vi "CRYSet Calibration Step to Calibrated Device.vi"(11 "Calibration setup In":string) -> (2 "output Calibration":T4 {"Calibration 2D"."Sens Curve"."Z data" items=["dB", "Lin"]; "Calibration 2D"."Sens Curve"."X data" items=["dB", "Lin"]; "Calibration 2D"."Sens Curve"."Y data" items=["dB", "Lin"]; "Calibration 2D"."Sens Curve"."Z dB ref" format="%.1f"; "Calibration 2D"."Sens Curve"."Z axis" items=["Log", "Lin"]; "Calibration 2D"."Sens Curve"."X dB ref" format="%.1f"; "Calibration 2D"."Sens Curve"."X axis" items=["Log", "Lin"]; "Calibration 2D"."Sens Curve"."Y axis" items=["Log", "Lin"]; "Calibration 2D"."Sens Curve"."Y dB ref" format="%.1f"; "Calibration 2D"."Sens Curve"."Curve"."z" format="%.2f"; "Calibration 2D"."Sens Curve"."Curve"."y" format="%.2f"; "Calibration 2D"."Sens Curve"."Curve"."x" format="%.2f"; "Calibration 2D"."EQ Curve"."Z data" items=["dB", "Lin"]; "Calibration 2D"."EQ Curve"."X data" items=["dB", "Lin"]; "Calibration 2D"."EQ Curve"."Y data" items=["dB", "Lin"]; "Calibration 2D"."EQ Curve"."Z dB ref" format="%.1f"; "Calibration 2D"."EQ Curve"."Z axis" items=["Log", "Lin"]; "Calibration 2D"."EQ Curve"."X dB ref" format="%.1f"; "Calibration 2D"."EQ Curve"."X axis" items=["Log", "Lin"]; "Calibration 2D"."EQ Curve"."Y axis" items=["Log", "Lin"]; "Calibration 2D"."EQ Curve"."Y dB ref" format="%.1f"; "Calibration 2D"."EQ Curve"."Curve"."z" format="%.2f"; "Calibration 2D"."EQ Curve"."Curve"."y" format="%.2f"; "Calibration 2D"."EQ Curve"."Curve"."x" format="%.2f"; "Calibration 2D"."Corr Curve"."Z data" items=["dB", "Lin"]; "Calibration 2D"."Corr Curve"."X data" items=["dB", "Lin"]; "Calibration 2D"."Corr Curve"."Y data" items=["dB", "Lin"]; "Calibration 2D"."Corr Curve"."Z dB ref" format="%.1f"; "Calibration 2D"."Corr Curve"."Z axis" items=["Log", "Lin"]; "Calibration 2D"."Corr Curve"."X dB ref" format="%.1f"; "Calibration 2D"."Corr Curve"."X axis" items=["Log", "Lin"]; "Calibration 2D"."Corr Curve"."Y axis" items=["Log", "Lin"]; "Calibration 2D"."Corr Curve"."Y dB ref" format="%.1f"; "Calibration 2D"."Corr Curve"."Curve"."z" format="%.2f"; "Calibration 2D"."Corr Curve"."Curve"."y" format="%.2f"; "Calibration 2D"."Corr Curve"."Curve"."x" format="%.2f"; "Calibration 2D"."Calibration"."EQ Step size" items=["R10", "R20", "R40", "R80", "User"]; "Calibration 2D"."Calibration"."Corr Step size" items=["R10", "R20", "R40", "R80", "User"]}, 3 "Calibration flattened out":string)   [LabVIEW 2013]
uses:
  Typedef Control/CRYCalibration All Cluster.ctl
  Typedef Control/CRYCalibration 2DCluster.ctl
  Typedef Control/CRYCalibration Cluster.ctl
  Typedef Control/CRYData Cluster.ctl
  CRYMainGlobal.vi
panel:
  in  "Calibration 2D":T1[](array[typedef]) {"Sens Curve"."Z data" items=["dB", "Lin"]; "Sens Curve"."X data" items=["dB", "Lin"]; "Sens Curve"."Y data" items=["dB", "Lin"]; "Sens Curve"."Z dB ref" format="%.1f"; "Sens Curve"."Z axis" items=["Log", "Lin"]; "Sens Curve"."X dB ref" format="%.1f"; "Sens Curve"."X axis" items=["Log", "Lin"]; "Sens Curve"."Y axis" items=["Log", "Lin"]; "Sens Curve"."Y dB ref" format="%.1f"; "Sens Curve"."Curve"."z" format="%.2f"; "Sens Curve"."Curve"."y" format="%.2f"; "Sens Curve"."Curve"."x" format="%.2f"; "EQ Curve"."Z data" items=["dB", "Lin"]; "EQ Curve"."X data" items=["dB", "Lin"]; "EQ Curve"."Y data" items=["dB", "Lin"]; "EQ Curve"."Z dB ref" format="%.1f"; "EQ Curve"."Z axis" items=["Log", "Lin"]; "EQ Curve"."X dB ref" format="%.1f"; "EQ Curve"."X axis" items=["Log", "Lin"]; "EQ Curve"."Y axis" items=["Log", "Lin"]; "EQ Curve"."Y dB ref" format="%.1f"; "EQ Curve"."Curve"."z" format="%.2f"; "EQ Curve"."Curve"."y" format="%.2f"; "EQ Curve"."Curve"."x" format="%.2f"; "Corr Curve"."Z data" items=["dB", "Lin"]; "Corr Curve"."X data" items=["dB", "Lin"]; "Corr Curve"."Y data" items=["dB", "Lin"]; "Corr Curve"."Z dB ref" format="%.1f"; "Corr Curve"."Z axis" items=["Log", "Lin"]; "Corr Curve"."X dB ref" format="%.1f"; "Corr Curve"."X axis" items=["Log", "Lin"]; "Corr Curve"."Y axis" items=["Log", "Lin"]; "Corr Curve"."Y dB ref" format="%.1f"; "Corr Curve"."Curve"."z" format="%.2f"; "Corr Curve"."Curve"."y" format="%.2f"; "Corr Curve"."Curve"."x" format="%.2f"; "Calibration"."EQ Step size" items=["R10", "R20", "R40", "R80", "User"]; "Calibration"."Corr Step size" items=["R10", "R20", "R40", "R80", "User"]}
  in  "Hz Out":dbl caption="Hz"
  in  "dB Out":dbl caption="Sensitivity" format="%#.2g"
  in  "Sens unit Out":string="V/V"
  out "EQ Curve Out":string caption="均等化曲线"
  out "dB ref Out":dbl=1.0 caption="dB参考" format="%#_3p"
  out "unit Out":string="V" caption="单位"
  in  "Sensitivity Out":dbl=1e-50 caption="感度" min=1e-50 format="%#_6p"
  out "Sens Value Out":string caption="感度值"
  out "Corre Curve Out":string caption="修正曲线"
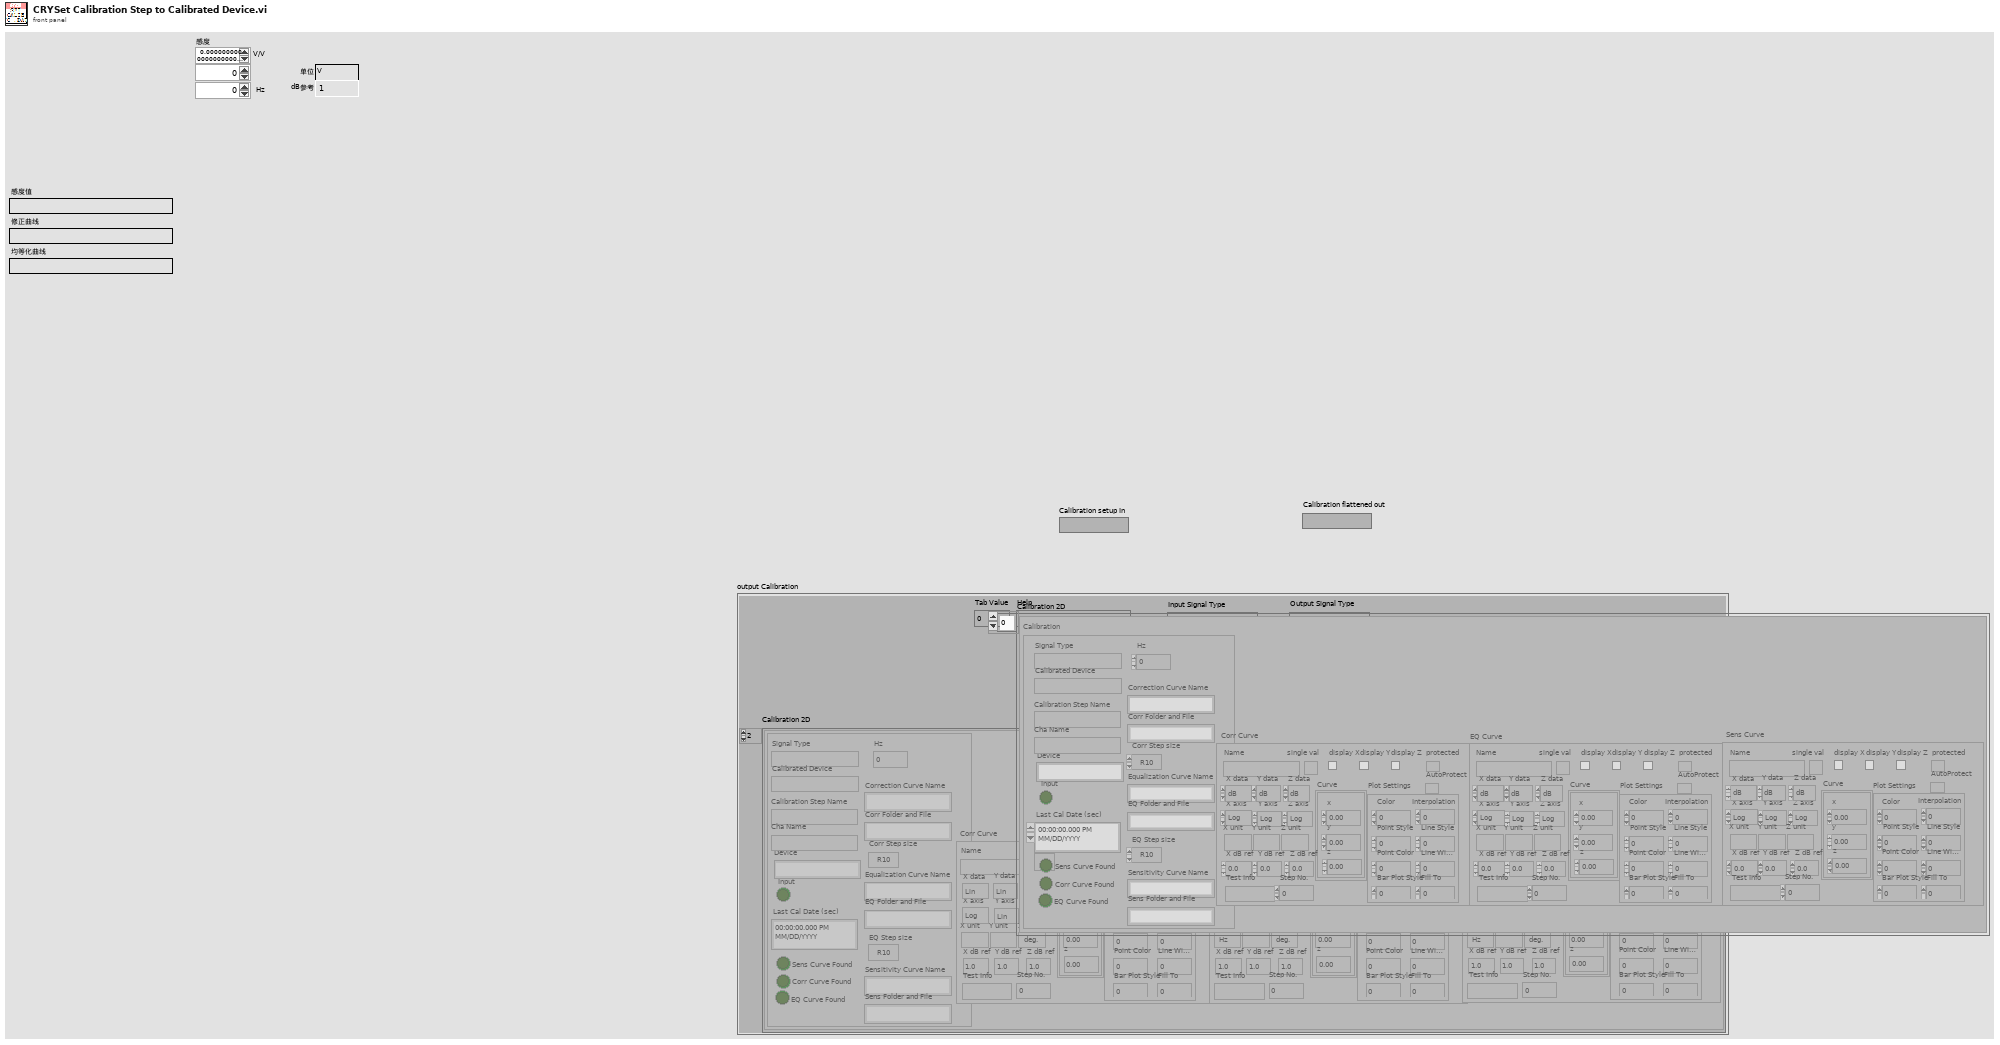
[diagram p1: front panel]
types:
  T1 = typedef "CRYCalibration 2DCluster.ctl" = cluster{"Calibration":T2, "Corr Curve":T3, "EQ Curve":T3, "Sens Curve":T3}
  T2 = typedef "CRYCalibration Cluster.ctl" = cluster{"Calibration Step Name":string, "Device":string, "Correction Curve Name":string, "Equalization Curve Name":string, "Sensitivity Curve Name":string, "Corr Folder and File":string, "EQ Folder and File":string, "Sens Folder and File":string, "Corr Step size":u16, "EQ Step size":u16, "Input":bool, "Last Cal Date (sec)":timestamp, "Cha Name":string, "Corr Curve Found":bool, "EQ Curve Found":bool, "Sens Curve Found":bool, "Signal Type":string, "Calibrated Device":string, "Hz":u32}
  T3 = typedef "CRYData Cluster.ctl" = cluster{"Name":string, "Curve":cluster{"x":dbl, "y":dbl, "z":dbl}[], "X data":u16, "Y data":u16, "Z data":u16, "X axis":u16, "Y axis":u16, "Z axis":u16, "X unit":string, "Y unit":string, "Z unit":string, "X dB ref":dbl, "Y dB ref":dbl, "Z dB ref":dbl, "single val":bool, "protected":bool, "display X":bool, "display Y":bool, "display Z":bool, "Test Info":string, "Step No.":i32, "Plot Settings":cluster{"Color":u32, "Interpolation":u8, "Point Style":u8, "Line Style":u8, "Point Color":u32, "Line Width":u8, "Bar Plot Style":u8, "Fill To":i16}, "AutoProtect":bool}
  T4 = typedef "CRYCalibration All Cluster.ctl" = cluster{"Calibration 2D":T1[], "Help":string, "Tab Value":i32, "Input Signal Type":string, "Output Signal Type":string}
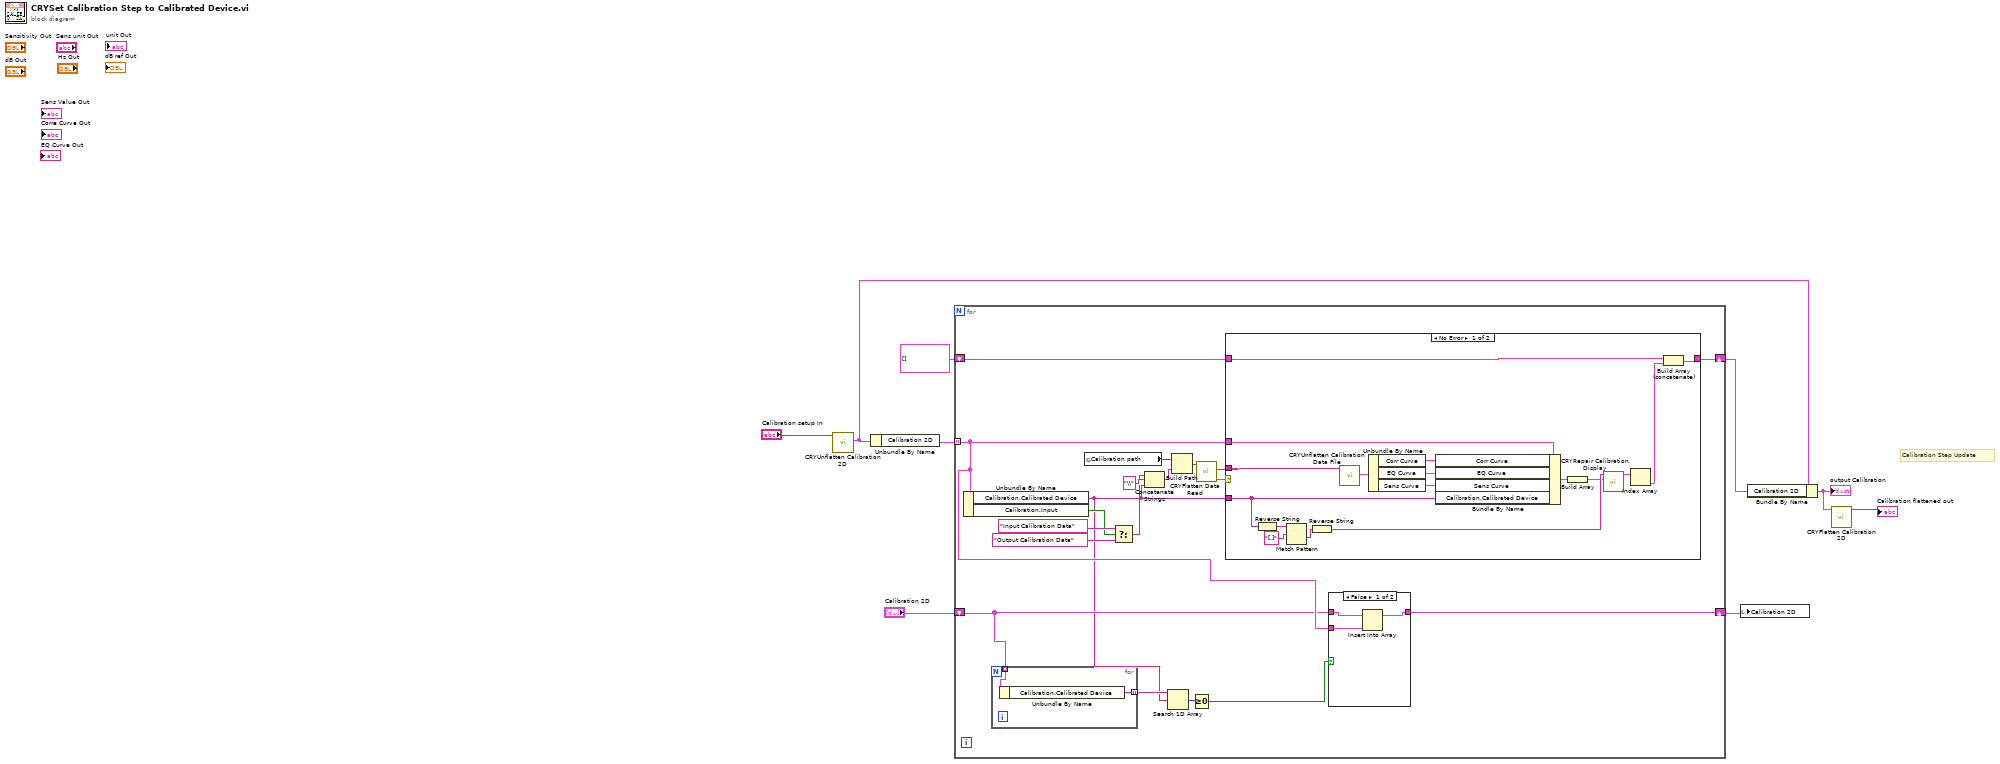
[diagram p0: block diagram]
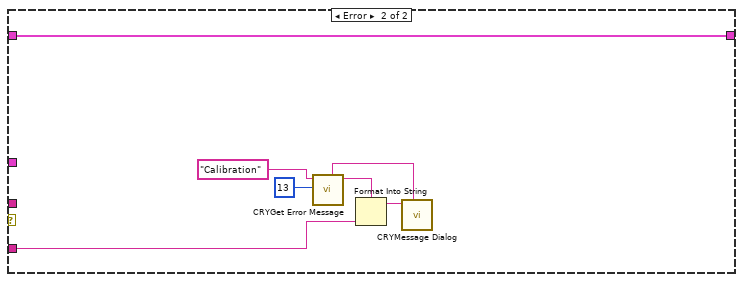
[diagram p3: hidden frame]
diagram:
  # "Calibration Step Update"
  n1 = call "CRYUnflatten Calibration 2D.vi"("Flattened Calibration"="Calibration setup In") -> ("Calibration Step Out"=w8:T4)  [unwired: 2 in, 8 out]
  n2 = Unbundle By Name(w8) -> ("Calibration 2D"=w9:T1[])
  n3 = for {
    tunnel: w9 -> [w15] mode=indexing
    shift-right: [w18] -> w4
    shift-left: T1[] [] -> [w19]
    shift-right: [w16] -> w1
    shift-left: "Calibration 2D" -> [w14]
    n4 = Unbundle By Name(w15) -> ("Calibration.Calibrated Device"=w12:string, "Calibration.Input"=w17:bool)
    n5 = for {
      tunnel: w14 -> [w34] mode=indexing
      tunnel: [w33] -> w13 mode=indexing
      n6 = Unbundle By Name(w34) -> ("Calibration.Calibrated Device"=w33:string)
    }
    n7 = global read "CRYMainGlobal.vi" "Calibration path"() -> (w22:path)
    n8 = Select(t="Input Calibration Data" ("name or relative path"), s=w17, f="Output Calibration Data" ("name or relative path")) -> (s? t:f=w20:string)
    n9 = Concatenate Strings(w20, "\\" ("string"), w12) -> (w25:string)
    n10 = Search 1D Array(1D array=w13, element=w12) -> (index of element=w11:i32)  [unwired: 1 in]
    n11 = Build Path(base path=w22, name or relative path=w25) -> (appended path=w23:path)
    n12 = Greater Or Equal To 0?(x=w11) -> (x >= 0?=w10:bool)
    n13 = call "CRYFlatten Data Read.vi"("Path In"=w23) -> ("error out"=w26:errorcluster, "Flatten Data Out"=w21:string)  [unwired: 6 in, 1 out]
    n14 = case shown="No Error" w26 {
      tunnel: w21 -> [w51 _]
      tunnel: w12 -> [w44 w52]
      tunnel: w15 -> [w38 _]
      tunnel: w19 -> [w37 w58]
      tunnel: [w35 w58] -> w18
      frame No Error {
        n15 = Reverse String(1:w44) -> (0:w43:string)
        n16 = Match Pattern(string=w43, regular expression="[.]") -> (after substring=w46:string)  [unwired: 4 out]
        n17 = Reverse String(1:w46) -> (0:w42:string)
        n18 = call "CRYUnflatten Calibration Data File.vi"("Flattened Calibration"=w51) -> ("Calibration 2D Data File Out"=w50:T1)  [unwired: 8 in, 2 out]
        n19 = Unbundle By Name(w50) -> ("Corr Curve"=w47:T3, "EQ Curve"=w48:T3, "Sens Curve"=w49:T3)
        n20 = Bundle By Name(cluster=w38, "Corr Curve"=w47, "EQ Curve"=w48, "Sens Curve"=w49, "Calibration.Calibrated Device"=w44) -> (w41:T1)
        n21 = Build Array(w41) -> (w40:T1[])
        n22 = call "CRYRepair Calibration Display.vi"("Calibration In"=w40, "Calibration Step Name"=w42) -> ("Calibration Out"=w39:T1[])  [unwired: 1 in, 8 out]
        n23 = Index Array(array=w39) -> (element=w36:T1)  [unwired: 1 in]
        n24 = Build Array (concatenate)(w37, w36) -> (w35:T1[])
      }
      frame Error {
        n25 = call "CRYGet Error Message.vi"("Error No"=13 ("No"), "Kind"="Calibration") -> ("Message"=w55:string, "Window Title"=w54:string)  [unwired: 4 in, 4 out]
        n26 = Format Into String(format string=w55, w52) -> (resulting string=w53:string)  [unwired: 2 in, 1 out]
        n27 = call "CRYMessage Dialog.vi"("Window Title"=w54, "Message Content"=w53) -> ()  [unwired: 8 in, 2 out]
      }
    }
    n28 = case shown="False" w10 {
      tunnel: w14 -> [w31 w32]
      tunnel: [w30 w32] -> w16
      tunnel: w15 -> [w29 _]
      frame False {
        n29 = Insert Into Array(array=w31, new element=w29) -> (w30:T1[])  [unwired: 1 in]
      }
      frame True {
      }
    }
  }
  n30 = local write "Calibration 2D"(w1) -> ()
  n31 = Bundle By Name(cluster=w8, "Calibration 2D"=w4) -> (w3:T4)
  "output Calibration" <- w3
  n32 = call "CRYFlatten Calibration 2D.vi"("Calibration All Cluster"=w3) -> ("Calibration flattened"=→"Calibration flattened out":string)  [unwired: 10 out]
